vi "Configure Trigger (RS232).vi"(0 "VISA resource name":refnum<visa-resource-name>, 1 "Baud Rate (9600)":i32=9600, 2 "Data Value":string, 5 "Data Source (0:Channel1)":u16(ring) items=["Channel1", "Channel2", "Channel3", "Channel4"], 7 "Data Threshold (1.0V)":dbl=1.0, 9 "Data Parity (0:ODD)":u16(ring) items=["Odd", "Even", "None"], 11 "error in (no error)":errorcluster) -> (4 "VISA resource name out":refnum<visa-resource-name>, 15 "error out":errorcluster)   [LabVIEW 2011, in "Tektronix 7000 Series.lvlib"]
doc: "Configures RS232 trigger settings for an oscilloscope.\n\nOnly DPO7000 series oscilloscopes support Serial Trigger."
uses:
  Tektronix 7000 Series.lvlib
panel:
  # "msb"
  # "lsb"
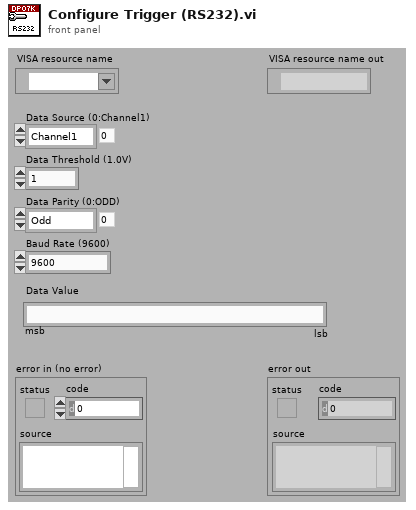
[diagram p1: front panel]
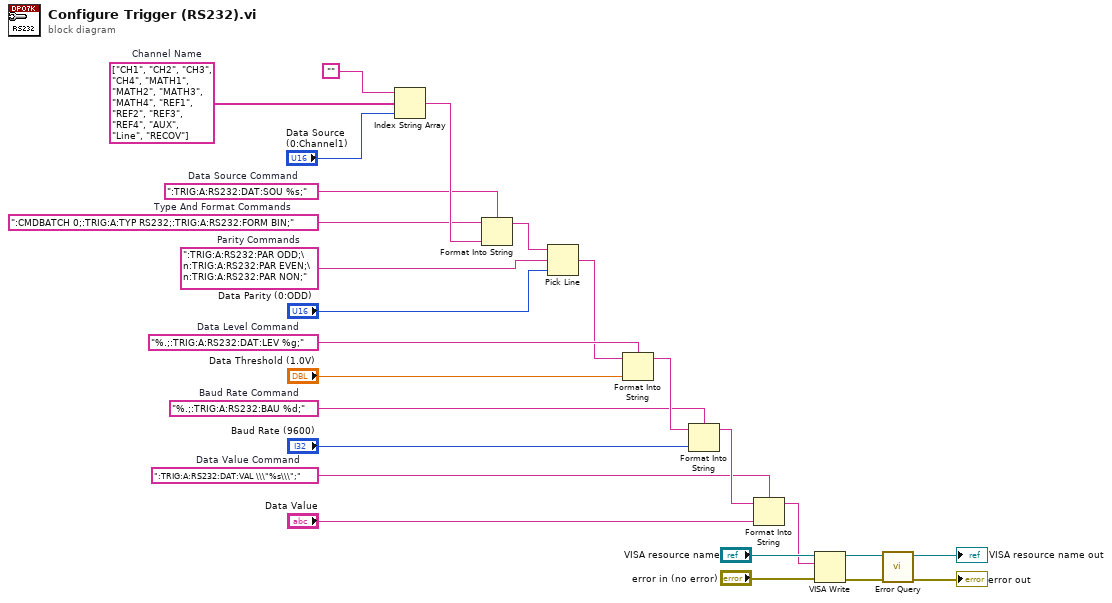
[diagram p0: block diagram]
diagram:
  w9 = ":TRIG:A:RS232:DAT:VAL \\\"%s\\\";"  # Data Value Command
  w11 = "%.;:TRIG:A:RS232:BAU %d;"  # Baud Rate Command
  w16 = "%.;:TRIG:A:RS232:DAT:LEV %g;"  # Data Level Command
  w19 = ":TRIG:A:RS232:PAR ODD;\n:TRIG:A:RS232:PAR EVEN;\n:TRIG:A:RS232:PAR NON;"  # Parity Commands
  w20 = ":TRIG:A:RS232:DAT:SOU %s;"  # Data Source Command
  w21 = ":CMDBATCH 0;:TRIG:A:TYP RS232;:TRIG:A:RS232:FORM BIN;"  # Type And Format Commands
  w25 = string[] ["CH1", "CH2", "CH3", "CH4", "MATH1", "MATH2", "MATH3", "MATH4", "REF1", "REF2", "REF3", "REF4", "AUX", "Line", "RECOV"]  # Channel Name
  n1 = Index String Array(1:"Data Source (0:Channel1)", 2:w25, 3:"") -> (0:w22:string)
  n2 = Format Into String(format string=w20, initial string=w21, w22) -> (resulting string=w18:string)  [unwired: 1 in, 1 out]
  n3 = Pick Line(string ("")=w18, multi-line string=w19, line index="Data Parity (0:ODD)") -> (output string=w14:string)
  n4 = Format Into String(format string=w16, initial string=w14, "Data Threshold (1.0V)") -> (resulting string=w12:string)  [unwired: 1 in, 1 out]
  n5 = Format Into String(format string=w11, initial string=w12, "Baud Rate (9600)") -> (resulting string=w10:string)  [unwired: 1 in, 1 out]
  n6 = Format Into String(format string=w9, initial string=w10, "Data Value") -> (resulting string=w1:string)  [unwired: 1 in, 1 out]
  n7 = VISA Write(VISA resource name="VISA resource name", write buffer=w1, error in (no error)="error in (no error)") -> (VISA resource name out=w6:refnum<visa-resource-name>, error out=w7:errorcluster)  [unwired: 1 out]
  n8 = call "Error Query.vi"("error in (no error)"=w7, "VISA resource name"=w6) -> ("error out"=→"error out":errorcluster, "VISA resource name out"=→"VISA resource name out":refnum<visa-resource-name>)  [unwired: 6 in, 2 out]
